vi "QTI Sensor Init.vi"(8 "error in (no error)":errorcluster) -> (0 "error out":errorcluster, 3 "Line Sensor":refnum<class "IIC.lvclass">)   [LabVIEW 2020]
uses:
  <vilib>/High Genius/HG_WSI_Tookit/Dependencies/Library/IIC/IIC.lvclass
  C:/Program Files (x86)/National Instruments/LabVIEW 2020/vi.lib/High Genius/HG_WSI_Tookit/Dependencies/Library/HG_LIB/HG_LIB.lvclass
  <vilib>/High Genius/HG_WSI_Tookit/Dependencies/Library/HG_LIB/HG_LIB.lvclass
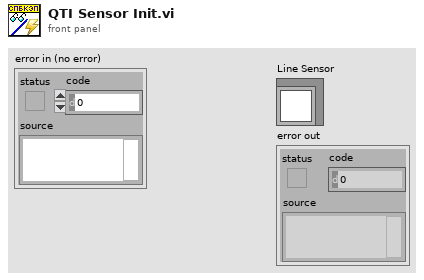
[diagram p1: front panel]
types:
  T1 = enum16{"DI", "DO", "AI", "Pulse", "PWM", "ISQ", "ENC", "CAN", "IIC", "IMU"}
  T2 = enum16{"0", "1", "2", "3", "4", "5", "6", "7", "8", "9", "10", "11", "12", "13", "14", "15", "16", "17", "18", "19", "20", "21", "22", "23", "24", "25"}
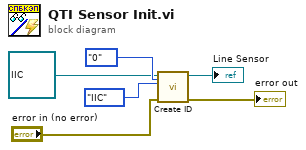
[diagram p0: block diagram]
diagram:
  n1 = call <vilib>:"Create ID.vi"("NO"=T2."0", "error in (no error)"="error in (no error)", "Function"=T1."IIC", "HG_LIB in"=refnum<class "IIC.lvclass"> refnum ("VMX Library.lvlib:IIC.lvclass")) -> ("error out"=→"error out":errorcluster, "HG_LIB out"=→"Line Sensor":refnum<class "IIC.lvclass">)  [unwired: 6 in]
